vi "Global_pid actif.vi"() -> ()   [LabVIEW 2014]
panel:
  out "ao0":dbl
  in  "pid temp?":bool=TRUE
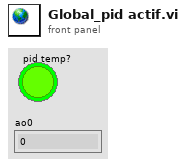
[diagram p1: front panel]
diagram:
